vi "Config File Name.vi"() -> (3 "Config File Name":string)   [LabVIEW 2020, in "SwerveDrive_ACT.lvlib"]
uses:
  roboRIO Code/Systems/SwerveDrive/SwerveDrive_ACT.lvlib
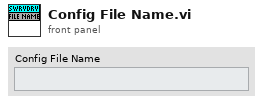
[diagram p1: front panel]
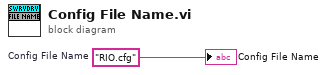
[diagram p0: block diagram]
diagram:
  w1 = "RIO.cfg"  # Config File Name
  "Config File Name" <- w1
